vi "Close File Do.vi"(8 "error in (no error)":errorcluster, 10 "File Path":path, 11 "TDMS File Writer in":refnum<class "File Writer_TDMS.lvclass">) -> (0 "error out":errorcluster, 3 "TDMS File Writer out":refnum<class "File Writer_TDMS.lvclass">)   [LabVIEW 2020, in "File Writer_TDMS.lvlib" / "File Writer_TDMS.lvclass"]
doc: "Close and defragment the TDMS file."
uses:
  File Writer_TDMS.lvclass
  File Writer_TDMS.lvclass/File Writer_TDMS.ctl
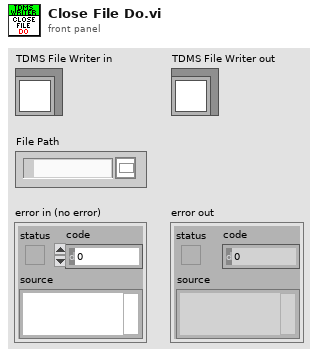
[diagram p1: front panel]
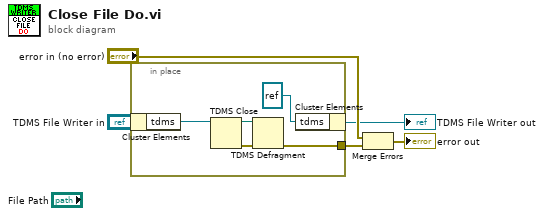
[diagram p0: block diagram]
diagram:
  n1 = in-place {
    in-place-border: [w8] -> w4
    n2 = in-place-cluster #1("TDMS File Writer in") -> ("tdms"=w6:refnum<k34>)
    n3 = TDMS Close(11:w6) -> (0:w9:errorcluster, 3:w10:path)  [unwired: 1 in]
    n4 = TDMS Defragment(4:w9, 7:w10) -> (0:w8:errorcluster)
    n5 = in-place-cluster #1("tdms"=refnum<k34> refnum) -> (→"TDMS File Writer out":refnum<class "File Writer_TDMS.lvclass">)
  }
  n6 = Merge Errors("error in (no error)", w4) -> (→"error out":errorcluster)
